vi "Open Sample Container Connections.vi"(8 "error in (no error)":errorcluster, 11 "Storage Line in":refnum<class "Storage Line.lvclass">) -> (0 "error out":errorcluster, 3 "Storage Line out":refnum<class "Storage Line.lvclass">)   [LabVIEW 2015, in "cRIO-Carbondioxide.lvlib" / "CO2-Actor.lvlib" / "Storage Line.lvclass"]
uses:
  Storage Line.lvclass
  Storage Line.lvclass/Storage Line.ctl
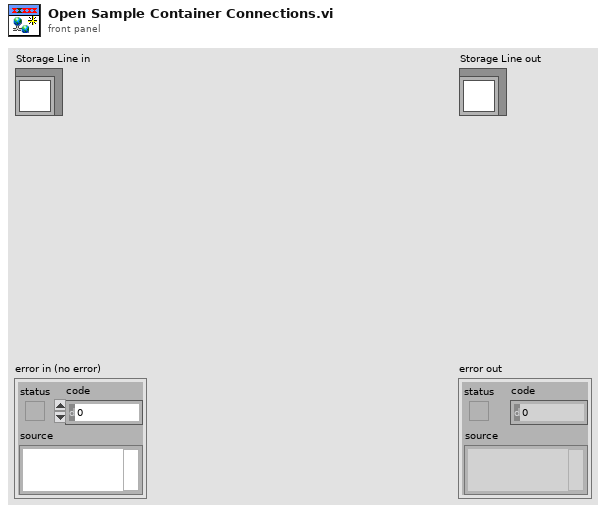
[diagram p1: front panel]
types:
  T1 = typedef "Sample Container.ctl" = cluster{"Sample In":refnum<k21>, "Sample Name":refnum<k21>, "Ti Cathode":refnum<k21>, "SampleQ":refnum<queue>}
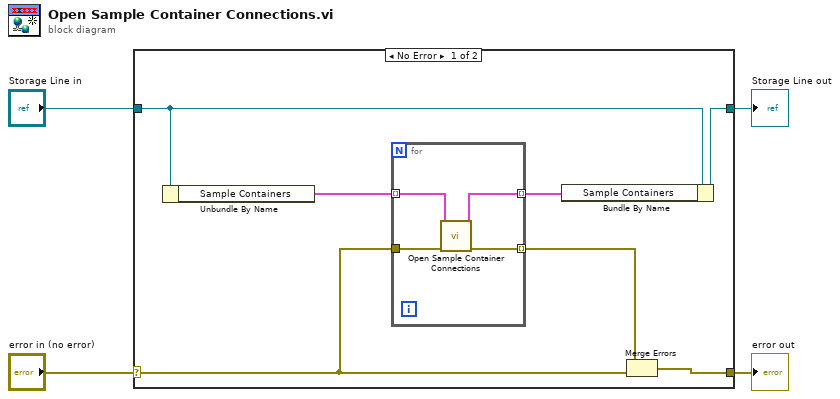
[diagram p0: block diagram]
diagram:
  n1 = case shown="No Error" "error in (no error)" {
    selector: "error in (no error)" -> [w9 w17]
    tunnel: [w8 w17] -> w3
    tunnel: [w6 w16] -> w1
    tunnel: "Storage Line in" -> [w11 w16]
    frame No Error {
      n2 = Unbundle By Name(w11) -> ("Sample Containers"=w10:T1[])
      n3 = for {
        tunnel: w10 -> [w14] mode=indexing
        tunnel: w9 -> [w15]
        tunnel: [w13] -> w5 mode=indexing
        tunnel: [w12] -> w7 mode=indexing
        n4 = call "Open Sample Container Connections.vi"("error in (no error)"=w15, "Container in"=w14) -> ("error out"=w12:errorcluster, "Container out"=w13:T1)  [unwired: 8 in]
      }
      n5 = Bundle By Name(cluster=w11, "Sample Containers"=w5) -> (w6:refnum<class "Storage Line.lvclass">)
      n6 = Merge Errors(w7, w9) -> (w8:errorcluster)
    }
    frame Error {
    }
  }
  "error out" <- w3
  "Storage Line out" <- w1
